vi "TwMass2Tof.vi"(1 "p":dbl[](array[numeric]), 2 "MassCalibMode":i32, 3 "Mass":dbl) -> (0 "TofSample":dbl)   [LabVIEW 2009]
uses:
  TwToolDll.dll
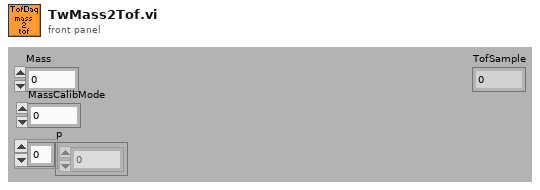
[diagram p1: front panel]
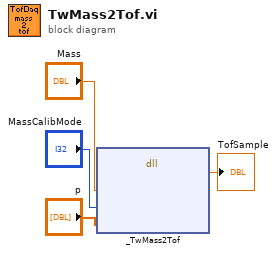
[diagram p0: block diagram]
diagram:
  n1 = dll-call lib="C:/src/TofDaq/APIandWrappers/LabView/TwToolDll/TwToolDll.dll" fn="_TwMass2Tof"("Mass"="Mass", "MassCalibMode"="MassCalibMode", "p"="p") -> ("TofSample"=→"TofSample":dbl)  [unwired: 6 in, 2 out]
